vi "RUN master.vi"   [LabVIEW 2016]
uses:
  <vilib>/NXT/Block Support/NXT_ButtonSelector.ctl
  <vilib>/NXT/Dual Mode Library/Waits/Wait_Btn_Press.vi
types:
  T1 = typedef "NXT_ButtonSelector.ctl" = u16
  T2 = typedef "LVHSConnector.ctl" = refnum<class "BrickReference.lvclass">
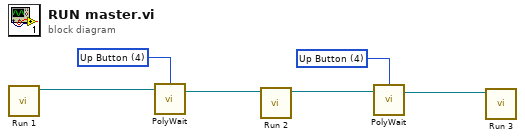
[diagram p0: block diagram]
diagram:
  w3 = T1 4 items=["Enter button"=3, "Left button"=2, "Right button"=1, "Up Button"=4, "Down Button"=5] ("Button (Enter button)")
  w5 = T1 4 items=["Enter button"=3, "Left button"=2, "Right button"=1, "Up Button"=4, "Down Button"=5] ("Button (Enter button)")
  n1 = call "Run 1.vi"() -> ("EV3 out"=w6:T2)  [unwired: 11 in]
  n2 = call-poly <vilib>:"PolyWait.vi"("NXT/EV3"=w6, "Button (Enter button)"=w5) -> ("NXT/EV3"=w4:T2)  [unwired: 2 in]
  n3 = call "Run 2.vi"("NXT/EV3"=w4) -> ("EV3 out"=w2:T2)  [unwired: 10 in]
  n4 = call-poly <vilib>:"PolyWait.vi"("NXT/EV3"=w2, "Button (Enter button)"=w3) -> ("NXT/EV3"=w1:T2)  [unwired: 2 in]
  n5 = call "Run 3.vi"("EV3 in"=w1) -> ()  [unwired: 10 in, 1 out]
